vi "boton.vi"(9 "error in (no error)":errorcluster, 10 "COM Bluegiga in":refnum<visa-resource-name>) -> (0 "error out":errorcluster, 1 "Numeric output":u8, 2 "Boolean output":bool, 3 "COM Bluegiga out":refnum<visa-resource-name>)   [LabVIEW 2020]
panel:
  out "characteristic value":u8[](array[numeric])
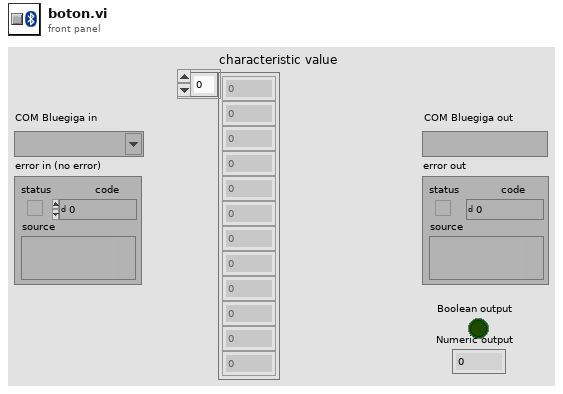
[diagram p1: front panel]
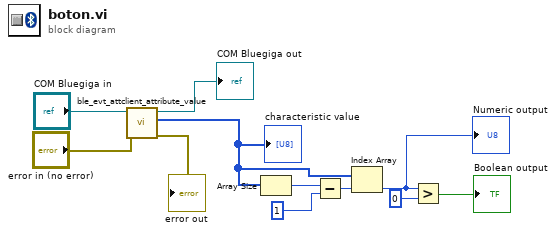
[diagram p0: block diagram]
diagram:
  n1 = call <vilib>:"ble_evt_attclient_attribute_value.vi"("error in (no error)"="error in (no error)", "COM Bluegiga in"="COM Bluegiga in") -> ("error out"=→"error out":errorcluster, "characteristic value"=w9:u8[], "COM Bluegiga out"=→"COM Bluegiga out":refnum<visa-resource-name>)  [unwired: 6 in, 1 out]
  "characteristic value" <- w9
  n2 = Array Size(array=w9) -> (size(s)=w8:i32)
  n3 = Subtract(x=w8, y=1) -> (x-y=w11:i32)
  n4 = Index Array(array=w9, index=w11) -> (element=w3:u8)
  "Numeric output" <- w3
  n5 = Greater?(x=w3, y=u8 0) -> (0:→"Boolean output":bool)
